vi "GetValue.vi"(8 "error in":errorcluster, 11 "Decimal in":refnum<class "Decimal.lvclass">) -> (0 "error out":errorcluster, 2 "Value":dbl, 3 "Decimal out":refnum<class "Decimal.lvclass">)   [LabVIEW 2021, in "ProligentXMLGenerator.lvlib" / "Decimal.lvclass"]
uses:
  Decimal.lvclass
  Decimal.lvclass/Decimal.ctl
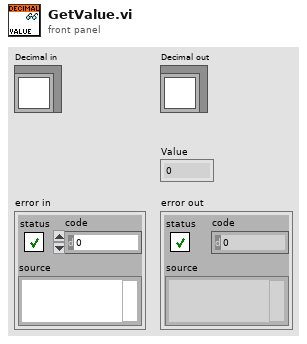
[diagram p1: front panel]
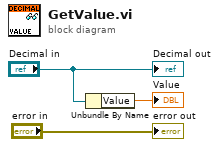
[diagram p0: block diagram]
diagram:
  n1 = Unbundle By Name("Decimal in") -> ("Value"=→"Value":dbl)
  "error out" <- "error in"
  "Decimal out" <- "Decimal in"
